vi "MeasurementSMO.GetPrivateEvents.vi"(8 "error in (no error)":errorcluster, 11 "MeasurementSMO":refnum<class "MeasurementSMO.lvclass">) -> (0 "error out":errorcluster, 2 "Private Events":T1, 3 "MeasurementSMO out":refnum<class "MeasurementSMO.lvclass">)   [LabVIEW 2019, in "MeasurementSMO.lvclass"]
doc: "---------------------------------------------------------------\nJKI State Machine Objects™\nhttp://jki.net/state-machine-objects/\nCopyright (C) 2005-2015, JKI <info@jki.net>\nALL RIGHTS RESERVEDJKI State Machine Objects (SMO) 1.0.0.4\nJKI - JKI\nCopyright (c) 2015, JKI"
uses:
  MeasurementSMO.lvclass
  Typedefs/PrivateEvents--Cluster.ctl
  Typedefs/PrivateEvents--MeasurementSMO.IV Run--Local.ctl
  Typedefs/PrivateEvents--MeasurementSMO.IV Status--Local.ctl
  MeasurementSMO.lvclass/MeasurementSMO.ctl
panel:
  # "For instructions on how to use the JKI State Machine Objects, examples and video tutorials, visit:\nhttp://jki.net/state-machine-objects/\n\nJKI State Machine Objects™\nhttp://jki.net/state-machine-objects/\nCopyright (C) 2005-2015, JKI <info@jki.net>\nALL RIGHTS RESERVED"
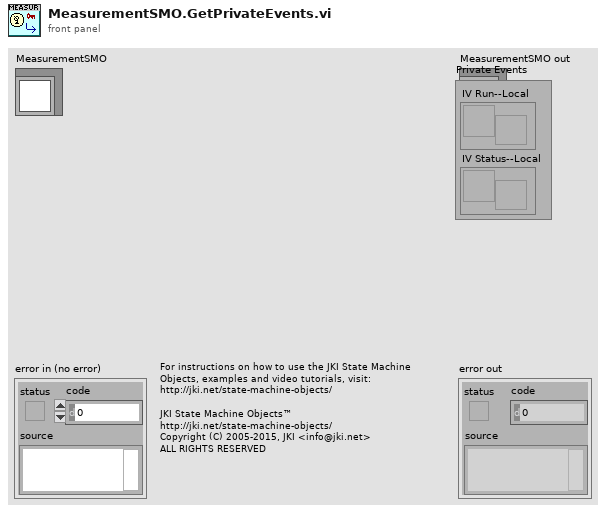
[diagram p1: front panel]
types:
  T1 = typedef "MeasurementSMO.lvclass/PrivateEvents--Cluster.ctl" = cluster{"IV Run--Local":refnum<user-event>, "IV Status--Local":refnum<user-event>}
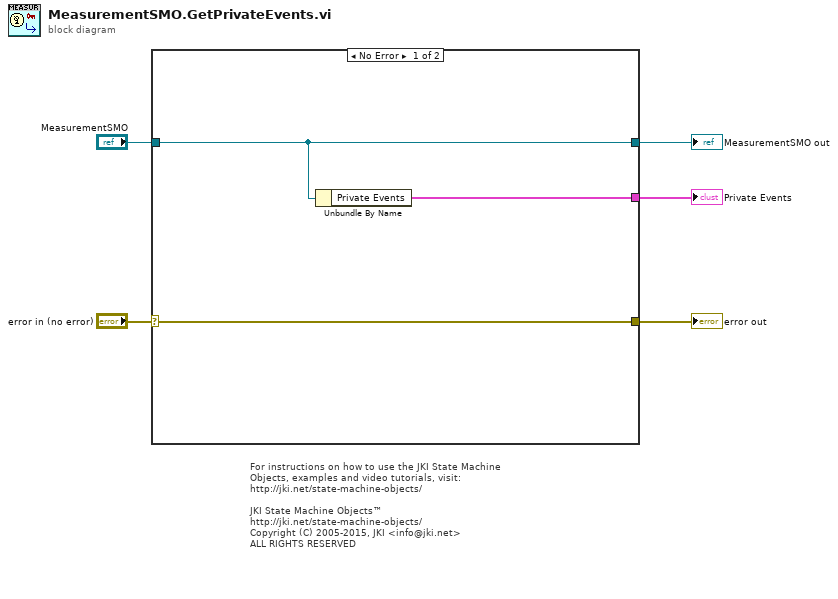
[diagram p0: block diagram]
diagram:
  # "For instructions on how to use the JKI State Machine Objects, examples and video tutorials, visit:\nhttp://jki.net/state-machine-objects/\n\nJKI State Machine Objects™\nhttp://jki.net/state-machine-objects/\nCopyright (C) 2005-2015, JKI <info@jki.net>\nALL RIGHTS RESERVED"
  n1 = case shown="No Error" "error in (no error)" {
    selector: "error in (no error)" -> [w7 w9]
    tunnel: "MeasurementSMO" -> [w6 w10]
    tunnel: [w7 w9] -> w4
    tunnel: [w6 w10] -> w3
    tunnel: [w8 _] -> w1
    frame No Error {
      n2 = Unbundle By Name(w6) -> ("Private Events"=w8:T1)
    }
    frame Error {
    }
  }
  "error out" <- w4
  "MeasurementSMO out" <- w3
  "Private Events" <- w1
